vi "Delete Service.vi"(8 "error in (no error)":errorcluster, 11 "Service in":refnum<class "Service.lvclass">) -> (0 "error out":errorcluster)   [LabVIEW 2024, in "Ramses Framework.lvlib" / "Service.lvclass"]
uses:
  Service.lvclass
  <vilib>/event_ctls.llb/usereventprio.ctl
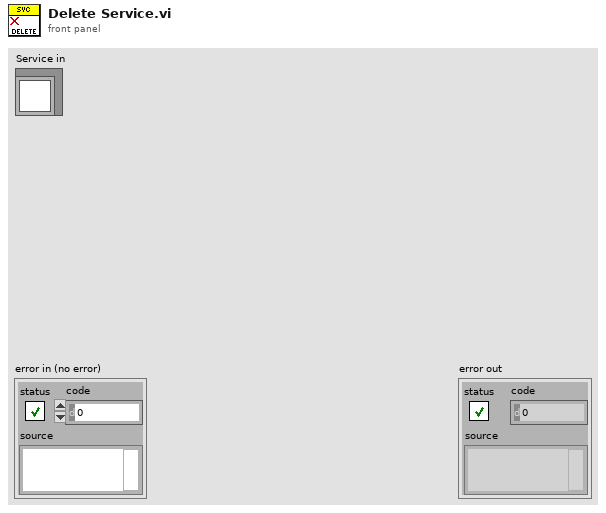
[diagram p1: front panel]
types:
  T1 = typedef "usereventprio.ctl" = enum32{"high priority", "normal priority"}
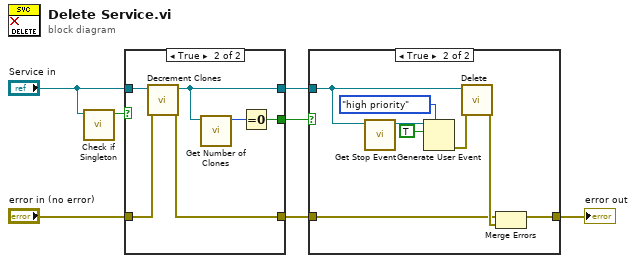
[diagram p0: block diagram]
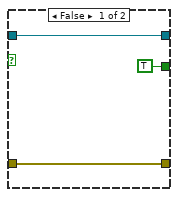
[diagram p2: hidden frame]
diagram:
  n1 = call-dynamic "Check if Singleton.vi"("Service in"="Service in") -> ("Singleton?"=w1:bool)  [unwired: 9 in, 1 out]
  n2 = case shown="True" w1 {
    tunnel: "Service in" -> [w10 w16]
    tunnel: [w10 w15] -> w5
    tunnel: [TRUE w13] -> w4
    tunnel: "error in (no error)" -> [w9 w12]
    tunnel: [w9 w11] -> w2
    frame False {
    }
    frame True {
      n3 = call "Decrement Clones.vi"("error in (no error)"=w12, "Service in"=w16) -> ("error out"=w11:errorcluster, "Service out"=w15:refnum<class "Service.lvclass">)  [unwired: 8 in]
      n4 = call "Get Number of Clones.vi"("Service in"=w15) -> ("Number of Clones"=w14:i32)  [unwired: 9 in, 1 out]
      n5 = Equal To 0?(x=w14) -> (x = 0?=w13:bool)
    }
  }
  n6 = case shown="True" w4 {
    tunnel: [w17 w24] -> w7
    tunnel: w2 -> [w17 w21]
    tunnel: w5 -> [_ w18]
    frame False {
    }
    frame True {
      n7 = call "Get Stop Event.vi"("Service in"=w18) -> ("Stop Event"=w23:refnum<user-event>)  [unwired: 9 in, 1 out]
      n8 = Generate User Event(priority (normal)=usereventprio."high priority", user event=w23, event data cluster=TRUE ("event data")) -> (error out=w20:errorcluster)  [unwired: 1 in, 1 out]
      n9 = call-dynamic "Delete.vi"("error in (no error)"=w20, "Service in"=w18) -> ("error out"=w25:errorcluster)  [unwired: 9 in]
      n10 = Merge Errors(w21, w25) -> (w24:errorcluster)
    }
  }
  "error out" <- w7
